vi "File_ListDirectory.vi"(0 "Directory Path":path, 1 "Treat LLB as directories?":bool, 3 "pattern (only dir)":string, 5 "error in (no error)":errorcluster, 6 "Reset":bool) -> (14 "Dup directory path":path, 15 "File names":string[](array[string]), 17 "Directory names":string[](array[string]), 18 "Top level":bool[](array[boolean]), 19 "error out":errorcluster)   [LabVIEW 2016]
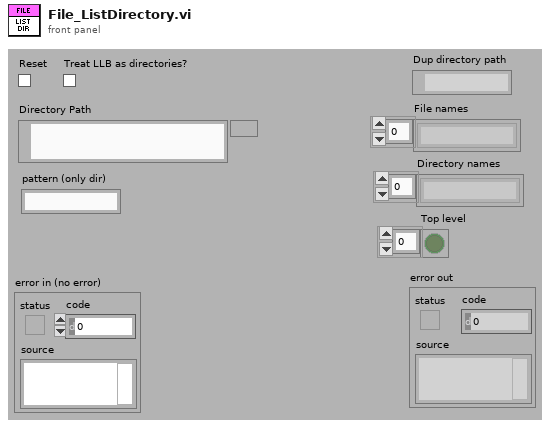
[diagram p1: front panel]
types:
  T1 = cluster{"File names":string[], "Directory names":string[], "Top level":bool[]}[]
  T2 = cluster{"File names out":string[], "Directory names out":string[], bool[]}
  T3 = cluster{"File names out":string[], "Directory names out":string[], "Top level":bool[]}[]
  T4 = typedef "Librarian File List.ctl" = cluster{"name":string, "create date":u32, "mod date":u32, "type":string, "creator":string, "LV version":i32}[]
  T5 = typedef "Librarian File Info Out.ctl" = cluster{"creation date":u32, "last mod date":u32, "type":string, "creator":string, "LV version":i32, "size":i32, "top level":bool}
  T6 = cluster{string[], "Directory names":string[], bool[]}
  T7 = cluster{"File names":string[], "Directory names":string[], "Top level":bool[]}
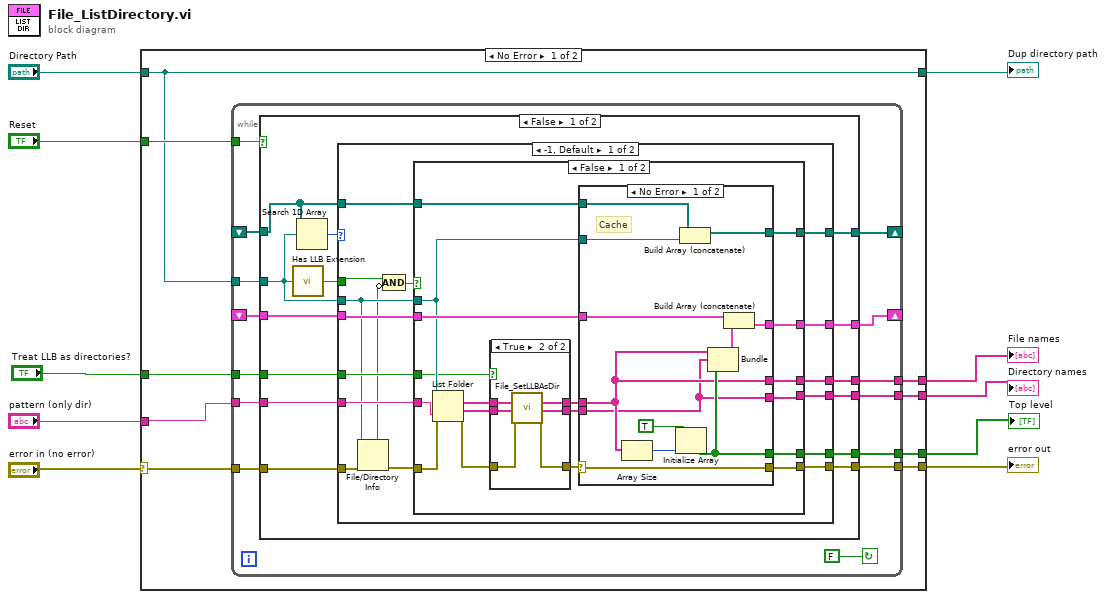
[diagram p0: block diagram]
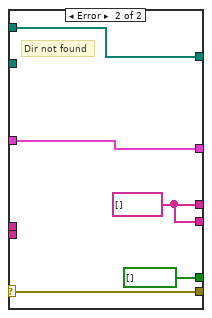
[diagram p2: hidden frame]
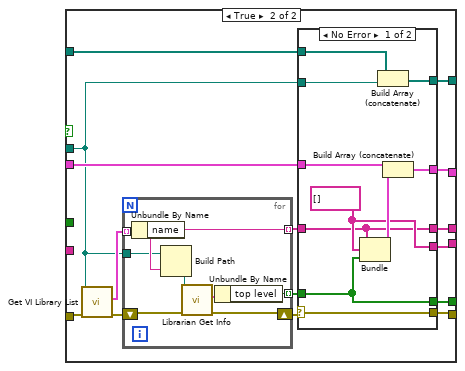
[diagram p4: hidden frame]
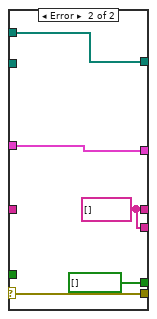
[diagram p5: hidden frame]
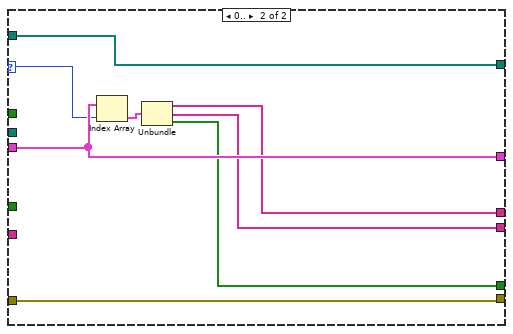
[diagram p6: hidden frame]
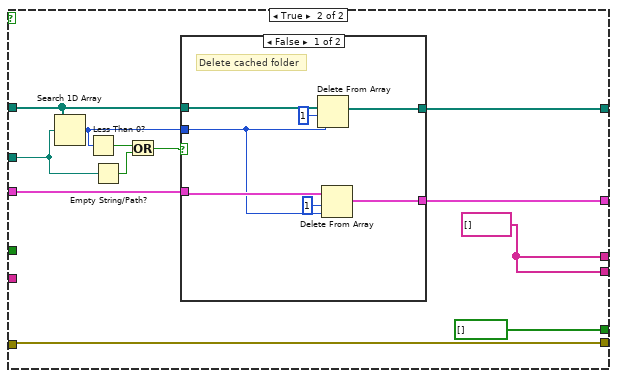
[diagram p7: hidden frame]
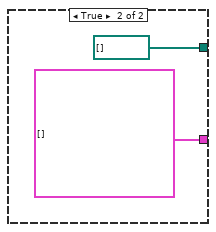
[diagram p8: hidden frame]
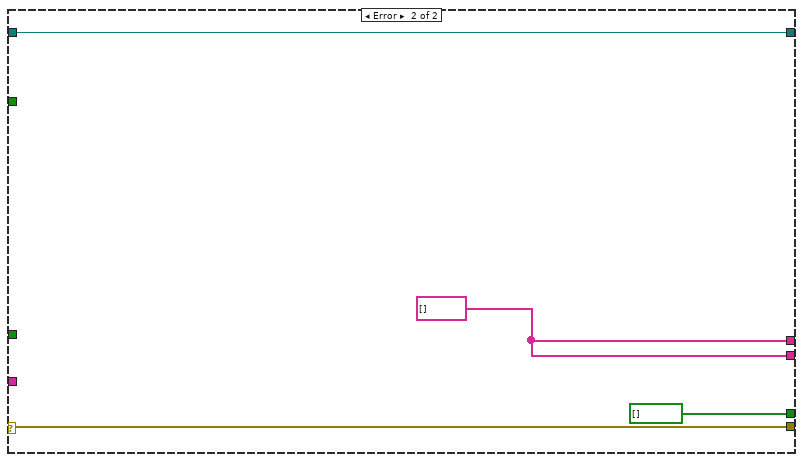
[diagram p9: hidden frame]
diagram:
  n1 = case shown="No Error" "error in (no error)" {
    selector: "error in (no error)" -> [w19 w177]
    tunnel: "Reset" -> [w18 _]
    tunnel: "Directory Path" -> [w15 w178]
    tunnel: "pattern (only dir)" -> [w13 _]
    tunnel: [w17 w176] -> w6
    tunnel: [w16 w176] -> w5
    tunnel: [w15 w178] -> w4
    tunnel: [w14 w177] -> w3
    tunnel: [w12 bool[] [] ("Top level")] -> w2
    tunnel: "Treat LLB as directories?" -> [w11 _]
    frame No Error {
      n2 = while {
        tunnel: w11 -> [w20]
        tunnel: [w21] -> w12
        tunnel: [w25] -> w14
        tunnel: w13 -> [w26]
        tunnel: [w29] -> w16
        tunnel: [w30] -> w17
        tunnel: w18 -> [w22]
        shift-left: _ -> [w23]
        shift-right: [w32] -> _
        shift-left: _ -> [w24]
        shift-right: [w31] -> _
        tunnel: w15 -> [w27]
        tunnel: w19 -> [w28]
        stop <- FALSE continue-if-true
        n3 = case shown="False" w22 {
          tunnel: [w46 w165] -> w32
          tunnel: [w45 w162] -> w31
          tunnel: [w44 w163] -> w30
          tunnel: [w43 w163] -> w29
          tunnel: w28 -> [w41 w164]
          tunnel: w27 -> [w40 w159]
          tunnel: w26 -> [w39 _]
          tunnel: [w38 w164] -> w25
          tunnel: w24 -> [w37 w155]
          tunnel: w23 -> [w36 w160]
          tunnel: [w35 bool[] []] -> w21
          tunnel: w20 -> [w34 _]
          frame False {
            n4 = call <vilib>:"Has LLB Extension.vi"("path"=w40) -> ("path to VI library?"=w42:bool)
            n5 = Search 1D Array(1D array=w36, element=w40) -> (index of element=w47:i32)  [unwired: 1 out]
            n6 = case shown="-1, Default" w47 {
              selector: w47 -> [_ w151]
              tunnel: w36 -> [w60 w153]
              tunnel: [w59 w153] -> w46
              tunnel: w37 -> [w62 w152]
              tunnel: [w61 w152] -> w45
              tunnel: [w57 w148] -> w44
              tunnel: [w56 w147] -> w43
              tunnel: w42 -> [w49 _]
              tunnel: w41 -> [w53 w150]
              tunnel: w40 -> [w51 _]
              tunnel: w39 -> [w63 _]
              tunnel: [w58 w150] -> w38
              tunnel: [w55 w146] -> w35
              tunnel: w34 -> [w54 _]
              frame -1, Default {
                n7 = File/Directory Info(path=w51, error in=w53) -> (directory=w50:bool, error out=w52:errorcluster)  [unwired: 5 out]
                n8 = Compound Arithmetic op=AND(w49, invert w50) -> (w48:bool)
                n9 = case shown="False" w48 {
                  tunnel: w52 -> [w81 w122]
                  tunnel: w51 -> [w76 w114]
                  tunnel: w63 -> [w75 _]
                  tunnel: w62 -> [w80 w120]
                  tunnel: [w79 w119] -> w61
                  tunnel: w60 -> [w78 w116]
                  tunnel: [w77 w117] -> w59
                  tunnel: [w68 w112] -> w58
                  tunnel: [w64 w110] -> w57
                  tunnel: [w66 w118] -> w56
                  tunnel: [w74 w109] -> w55
                  tunnel: w54 -> [w71 _]
                  frame False {
                    n10 = List Folder(path=w76, pattern=w75, error in=w81) -> (filenames=w73:string[], folder names=w72:string[], error out=w70:errorcluster)  [unwired: 2 out]
                    n11 = case shown="True" w71 {
                      tunnel: [w99 w106] -> w69
                      tunnel: w73 -> [w101 w105]
                      tunnel: w72 -> [w100 w104]
                      tunnel: [w101 w103] -> w65
                      tunnel: [w100 w102] -> w67
                      tunnel: w70 -> [w99 w107]
                      frame False {
                      }
                      frame True {
                        n12 = call <resource>:"File_SetLLBAsDir.vi"("File names"=w105, "Directory names"=w104, "error in (no error)"=w107) -> ("File names out"=w103:string[], "Directory names out"=w102:string[], "error out"=w106:errorcluster)  [unwired: 14 out]
                      }
                    }
                    n13 = case shown="No Error" w69 {
                      selector: w69 -> [w84 w96]
                      tunnel: w80 -> [w93 w97]
                      tunnel: [w91 w97] -> w79
                      tunnel: w78 -> [w90 w98]
                      tunnel: [w89 w98] -> w77
                      tunnel: w76 -> [w88 _]
                      tunnel: [w85 bool[] []] -> w74
                      tunnel: w65 -> [w83 _]
                      tunnel: w67 -> [w82 _]
                      tunnel: [w84 w96] -> w68
                      tunnel: [w82 w94] -> w66
                      tunnel: [w83 w94] -> w64
                      frame No Error {
                        # "Cache"
                        n14 = Array Size(array=w83) -> (size(s)=w87:i32)
                        n15 = Initialize Array(TRUE, w87) -> (w85:bool[])
                        n16 = Build Array (concatenate)(w90, w88) -> (w89:path[])
                        n17 = Bundle("File names out"=w83, "Directory names out"=w82, w85) -> (w92:T2)  [unwired: 1 out]
                        n18 = Build Array (concatenate)(w93, w92) -> (w91:T3)
                      }
                      frame Error {
                        w94 = string[] []
                        # "Dir not found"
                      }
                    }
                  }
                  frame True {
                    n19 = call <vilib>:"Get VI Library List.vi"("error in (no error)"=w122, "library path"=w114) -> ("error out"=w115:errorcluster, "file list"=w121:T4)  [unwired: 8 out]
                    n20 = for {
                      tunnel: w121 -> [w145] mode=indexing
                      tunnel: [w141] -> w111 mode=indexing
                      shift-right: [w143] -> w113
                      shift-left: w115 -> [w144]
                      tunnel: w114 -> [w140]
                      tunnel: [w138] -> w108 mode=indexing
                      n21 = Unbundle By Name(w145) -> ("name"=w141:string)
                      n22 = Build Path(base path=w140, name or relative path=w141) -> (appended path=w142:path)
                      n23 = call <vilib>:"Librarian Get Info.vi"("error in (no error)"=w144, "path"=w142) -> ("error out"=w143:errorcluster, "file information"=w139:T5)  [unwired: 8 out]
                      n24 = Unbundle By Name(w139) -> ("top level"=w138:bool)
                    }
                    n25 = case shown="No Error" w113 {
                      selector: w113 -> [w125 w135]
                      tunnel: w120 -> [w132 w136]
                      tunnel: [w131 w136] -> w119
                      tunnel: [w129 w134] -> w118
                      tunnel: w111 -> [w124 _]
                      tunnel: [w128 w137] -> w117
                      tunnel: w116 -> [w127 w137]
                      tunnel: w114 -> [w126 _]
                      tunnel: w108 -> [w123 _]
                      tunnel: [w125 w135] -> w112
                      tunnel: [w124 w134] -> w110
                      tunnel: [w123 bool[] []] -> w109
                      frame No Error {
                        w129 = string[] [] ("Directory names")
                        n26 = Bundle(w124, "Directory names"=w129, w123) -> (w130:T6)  [unwired: 1 out]
                        n27 = Build Array (concatenate)(w127, w126) -> (w128:path[])
                        n28 = Build Array (concatenate)(w132, w130) -> (w131:T1)
                      }
                      frame Error {
                        w134 = string[] []
                      }
                    }
                  }
                }
              }
              frame 0.. {
                n29 = Index Array(array=w152, index=w151) -> (element=w149:T7)
                n30 = Unbundle(w149) -> ("File names"=w148:string[], "Directory names"=w147:string[], "Top level"=w146:bool[])
              }
            }
          }
          frame True {
            w163 = string[] [] ("file names")
            n31 = Search 1D Array(1D array=w160, element=w159) -> (index of element=w154:i32)  [unwired: 1 out]
            n32 = Less Than 0?(x=w154) -> (x < 0?=w157:bool)
            n33 = Empty String/Path?(string/path=w159) -> (empty?=w158:bool)
            n34 = Or(x=w157, y=w158) -> (x .or. y?=w156:bool)
            n35 = case shown="False" w156 {
              tunnel: [w171 path[] [] ("Array Constant")] -> w165
              tunnel: [w167 T1 [] ("Array Constant")] -> w162
              tunnel: w160 -> [w172 _]
              tunnel: w155 -> [w168 _]
              tunnel: w154 -> [w166 _]
              frame False {
                # "Delete cached folder"
                n36 = Delete From Array(array=w172, length=1 ("Length"), index=w166) -> (array with subset deleted=w171:path[])  [unwired: 1 out]
                n37 = Delete From Array(array=w168, length=1 ("Length"), index=w166) -> (array with subset deleted=w167:T1)  [unwired: 1 out]
              }
              frame True {
              }
            }
          }
        }
      }
    }
    frame Error {
      w176 = string[] []
    }
  }
  "File names" <- w6
  "Directory names" <- w5
  "error out" <- w3
  "Dup directory path" <- w4
  "Top level" <- w2
